vi "Page_Source_Top_Supports_Multiple_Items.vi"(8 "error in (no error)":errorcluster, 11 "AB_Build in":refnum<class "AB_Build.lvclass">) -> (0 "error out":errorcluster, 2 "multiple items":bool, 3 "AB_Build out":refnum<class "AB_Build.lvclass">)   [LabVIEW 2020, in "AB_Build.lvclass"]
uses:
  <vilib>/AppBuilder/AB_Classes/Build/AB_Build.lvclass
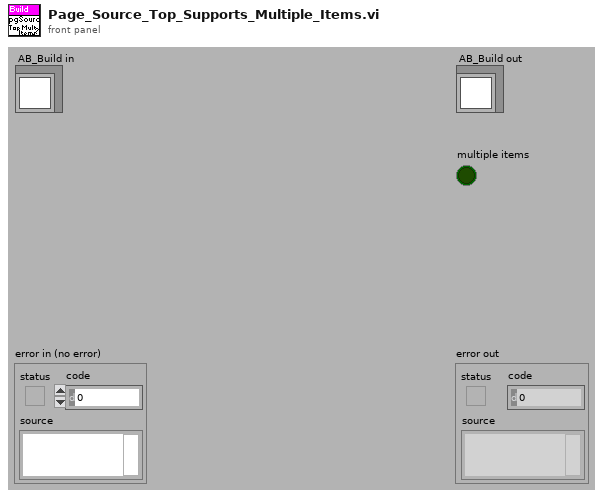
[diagram p1: front panel]
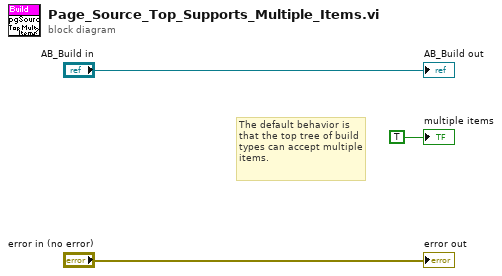
[diagram p0: block diagram]
diagram:
  # "The default behavior is that the top tree of build types can accept multiple items."
  "error out" <- "error in (no error)"
  "AB_Build out" <- "AB_Build in"
  "multiple items" <- TRUE ("canAddToTop")
